vi "Read Signal Generator 1.lvclass.vi"(11 "IMD in":refnum<class "IMD.lvclass">) -> (2 "Signal Generator 1.lvclass":refnum<class "Signal Generator.lvclass">, 3 "IMD out":refnum<class "IMD.lvclass">)   [LabVIEW 2020, in "IMD.lvclass"]
uses:
  IMD.lvclass
  Instruments/Signal Generator/Signal Generator.lvclass
  IMD.lvclass/IMD.ctl
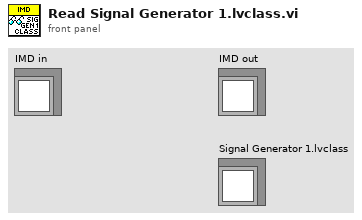
[diagram p1: front panel]
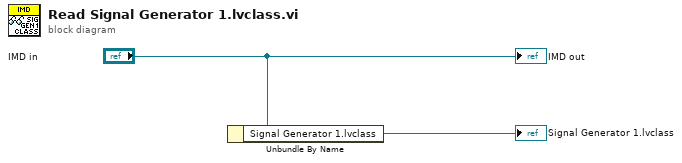
[diagram p0: block diagram]
diagram:
  n1 = Unbundle By Name("IMD in") -> ("Signal Generator 1.lvclass"=→"Signal Generator 1.lvclass":refnum<class "Signal Generator.lvclass">)
  "IMD out" <- "IMD in"
